vi "LogIntFloatTelemParam (SubVI).vi"(8 "error in":errorcluster, 11 "ArrayData":T1) -> (0 "error out":errorcluster)   [LabVIEW 2017]
uses:
  LV_Unicorn/Control/unicorn_array.ctl
  LV_Unicorn/LV_Unicorn.lvlib
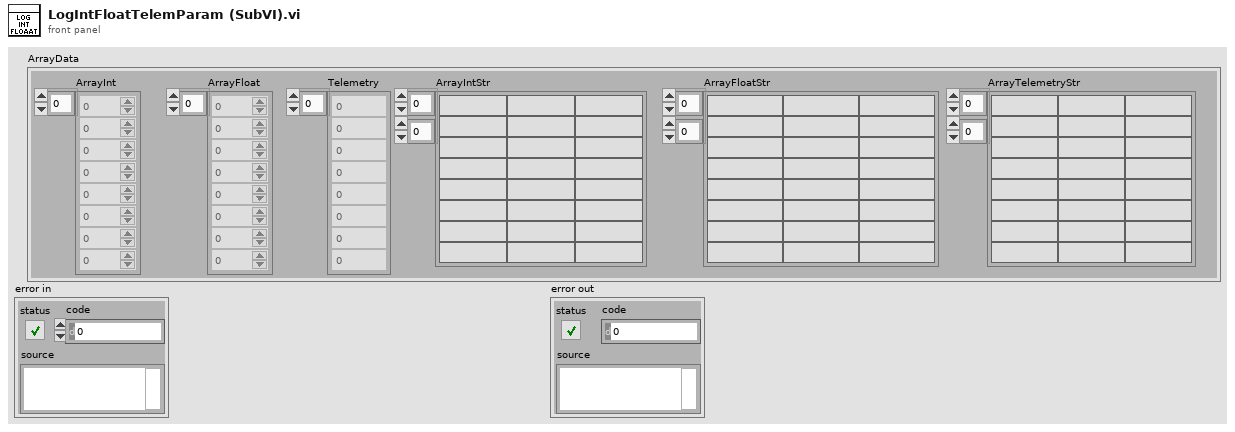
[diagram p1: front panel]
types:
  T1 = typedef "LV_Unicorn.lvlib/unicorn_array.ctl" = cluster{"ArrayInt":i32[], "ArrayFloat":sgl[], "Telemetry":sgl[], "ArrayIntStr":string[][], "ArrayFloatStr":string[][], "ArrayTelemetryStr":string[][]}
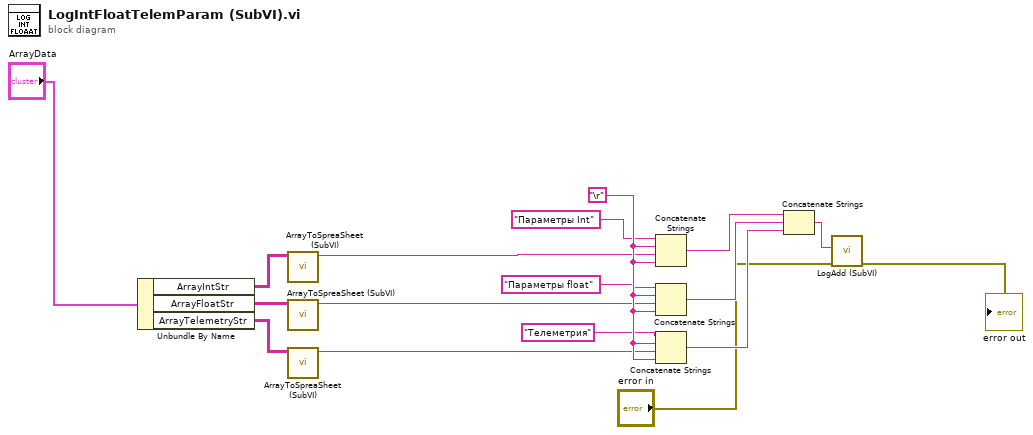
[diagram p0: block diagram]
diagram:
  w13 = "\r"
  n1 = Unbundle By Name("ArrayData") -> ("ArrayIntStr"=w14:string[][], "ArrayFloatStr"=w15:string[][], "ArrayTelemetryStr"=w16:string[][])
  n2 = call "ArrayToSpreaSheet (SubVI).vi"("ArrayTelemetryStr"=w14) -> ("spreadsheet string"=w12:string)  [unwired: 10 in]
  n3 = call "ArrayToSpreaSheet (SubVI).vi"("ArrayTelemetryStr"=w15) -> ("spreadsheet string"=w11:string)  [unwired: 10 in]
  n4 = call "ArrayToSpreaSheet (SubVI).vi"("ArrayTelemetryStr"=w16) -> ("spreadsheet string"=w10:string)  [unwired: 10 in]
  n5 = Concatenate Strings("Параметры Int" ("string"), w13, w12, w13) -> (w3:string)
  n6 = Concatenate Strings("Параметры float" ("string"), w13, w11, w13) -> (w4:string)
  n7 = Concatenate Strings("Телеметрия" ("string"), w13, w10, w13) -> (w5:string)
  n8 = Concatenate Strings(w3, w4, w5) -> (w6:string)
  n9 = call "LogAdd (SubVI).vi"("error in"="error in", "string"=w6) -> ("error out"=→"error out":errorcluster)  [unwired: 9 in]
